vi "Read Message.vi"(6 "timeout in ms (100)":i32=100, 8 "error in (no error)":errorcluster, 10 "index":i32, 11 "RemoteControl.ZMQ in":refnum<class "RemoteControl.ZMQ.lvclass">) -> (0 "error out":errorcluster, 1 "Data":variant, 2 "Command":string, 3 "RemoteControl.ZMQ out":refnum<class "RemoteControl.ZMQ.lvclass">, 4 "Message ID":i32)   [LabVIEW 2016, in "RemoteControl.ZMQ.lvclass"]
uses:
  RemoteControl.ZMQ.lvclass
  <vilib>/addons/zeromq/zmq_socket.lvclass
  RemoteControl/Typedefs/Message--Cluster.ctl
  RemoteControl/RemoteControl.lvclass
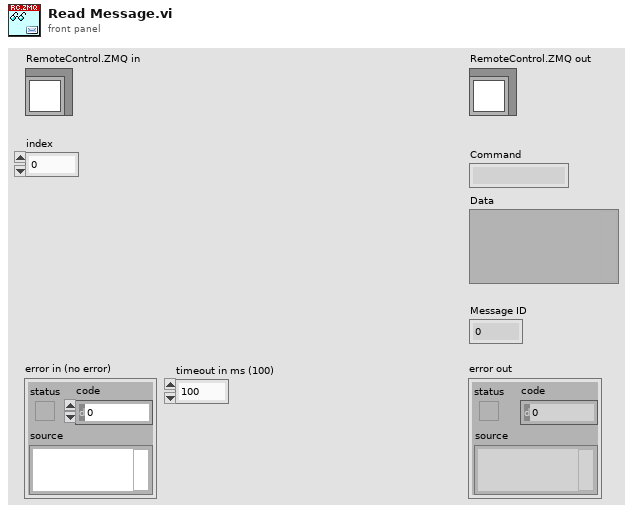
[diagram p1: front panel]
types:
  T1 = typedef "RemoteControl.lvclass/Message--Cluster.ctl" = cluster{"Command":string, "Data":variant, "Message ID":i32}
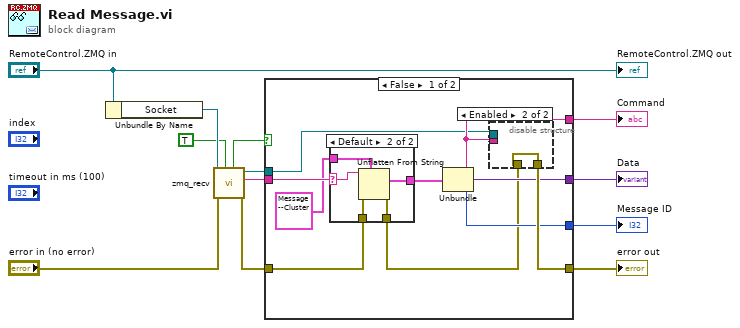
[diagram p0: block diagram]
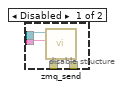
[diagram p2: hidden frame]
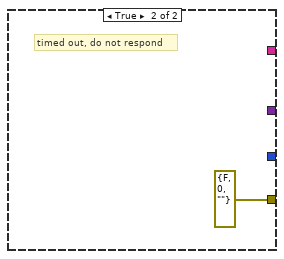
[diagram p4: hidden frame]
diagram:
  n1 = Unbundle By Name("RemoteControl.ZMQ in") -> ("Socket"=w10:refnum<class "zmq_socket.lvclass">)
  n2 = call <vilib>:"zmq_recv.vi"("no block? (F)"=TRUE, "error in"="error in (no error)", "socket in"=w10) -> ("error out"=w4:errorcluster, "data"=w2:string, "socket out"=w3:refnum<class "zmq_socket.lvclass">, "timeout?"=w1:bool)  [unwired: 2 in, 1 out]
  n3 = case shown="False" w1 {
    tunnel: [w22 errorcluster {"status"=FALSE, "code"=0, "source"=""} ("error out")] -> w11
    tunnel: [w21 _] -> w9
    tunnel: [w20 _] -> w8
    tunnel: [w19 _] -> w6
    tunnel: w4 -> [w17 _]
    tunnel: w3 -> [w15 _]
    tunnel: w2 -> [w14 _]
    frame False {
      n4 = case shown="Default" w14 {
        selector: w14 -> [_ w30]
        tunnel: T1 {"Command"="", "Data"=variant, "Message ID"=0} ("Message") -> [w28 w31]
        tunnel: [w28 w34] -> w18
        tunnel: w17 -> [w29 w33]
        tunnel: [w29 w32] -> w16
        frame "" {
        }
        frame Default {
          n5 = Unflatten From String(type=w31, binary string=w30, error in (no error)=w33) -> (value=w34:T1, error out=w32:errorcluster)  [unwired: 2 in, 1 out]
        }
      }
      n6 = Unbundle(w18) -> ("Command"=w19:string, "Data"=w21:variant, "Message ID"=w20:i32)
      n7 = disable-structure shown="Enabled" {
        disable-tunnel: [w26 w27] -> w22
        disable-tunnel: w19 -> [w25 _]
        disable-tunnel: w16 -> [w24 w27]
        disable-tunnel: w15 -> [w23 _]
        frame Disabled {
          n8 = call <vilib>:"zmq_send.vi"("error in"=w24, "data"=w25, "socket in"=w23) -> ("error out"=w26:errorcluster)  [unwired: 4 in, 1 out]
        }
        frame Enabled {
        }
      }
    }
    frame True {
      # "timed out, do not respond"
    }
  }
  "error out" <- w11
  "Message ID" <- w8
  "Command" <- w6
  "Data" <- w9
  "RemoteControl.ZMQ out" <- "RemoteControl.ZMQ in"
